vi "Build Instruction List.vi"(6 "Instruction List Starting Offset":u16=2048 format="%04x", 7 "Virtual Memory Unit in":refnum<class "Virtual Memory Unit.lvclass">, 8 "error in (no error)":errorcluster, 11 "Bus Controller in":refnum<class "Bus Controller.lvclass">) -> (0 "error out":errorcluster, 3 "Bus Controller out":refnum<class "Bus Controller.lvclass">, 4 "Instruction List Final Address":u16=2048 format="%04x", 5 "Virtual Memory Unit out":refnum<class "Virtual Memory Unit.lvclass">)   [LabVIEW 2020, in "BCI-1553 API.lvlib" / "Bus Controller.lvclass"]
doc: "Builds the entire instruction list that this Bus Controller will usefor data transactions. The Major Frame must be configured and constructed correctly for this procedure to operate as intended."
uses:
  Bus Controller.lvclass
  Dependencies/Virtual Memory Unit/Virtual Memory Unit.lvclass
  Bus Controller.lvclass/Bus Controller.ctl
  Frames & Messages/Major Frame/Major Frame.lvclass
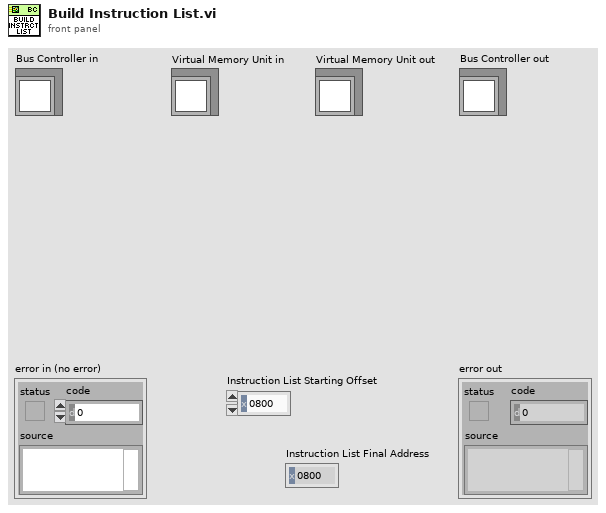
[diagram p1: front panel]
types:
  T1 = cluster{"HP Async Check Addresses":u16[], "HP Async Control Addresses":u16[], "HP Async Data Addresses":u16[], "LP Async Check Addresses":u16[], "LP Async Control Addresses":u16[], "LP Async Data Addresses":u16[]}
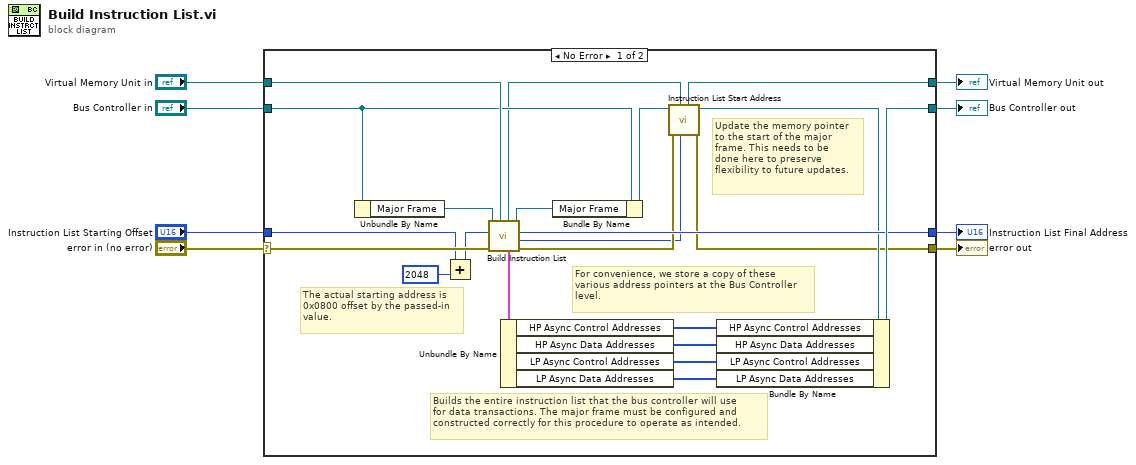
[diagram p0: block diagram]
diagram:
  n1 = case shown="No Error" "error in (no error)" {
    selector: "error in (no error)" -> [w26 w34]
    tunnel: [w15 w34] -> w7
    tunnel: [w20 w33] -> w5
    tunnel: "Bus Controller in" -> [w27 w33]
    tunnel: "Virtual Memory Unit in" -> [w29 w32]
    tunnel: [w12 w32] -> w3
    tunnel: "Instruction List Starting Offset" -> [w10 w31]
    tunnel: [w19 w31] -> w1
    frame No Error {
      # "The actual starting address is\n0x0800 offset by the passed-in\nvalue."
      # "Update the memory pointer\nto the start of the major\nframe. This needs to be\ndone here to preserve\nflexibility to future updates."
      # "For convenience, we store a copy of these\nvarious address pointers at the Bus Controller\nlevel."
      # "Builds the entire instruction list that the bus controller will use\nfor data transactions. The major frame must be configured and\nconstructed correctly for this procedure to operate as intended."
      n2 = Unbundle By Name(w27) -> ("Major Frame"=w30:refnum<class "Major Frame.lvclass">)
      n3 = Add(x=w10, y=u16 2048) -> (x+y=w9:u16)
      n4 = call-dynamic "Build Instruction List.vi"("Virtual Memory Unit in"=w29, "error in (no error)"=w26, "Starting Address"=w9, "Major Frame in"=w30) -> ("error out"=w16:errorcluster, "Instruction List Starting Address"=w14:u16, "Next Available Address"=w19:u16, "Major Frame out"=w28:refnum<class "Major Frame.lvclass">, "Async Pointers"=w25:T1, "Virtual Memory Unit out"=w13:refnum<class "Virtual Memory Unit.lvclass">)  [unwired: 2 in]
      n5 = Unbundle By Name(w25) -> ("HP Async Control Addresses"=w24:u16[], "HP Async Data Addresses"=w23:u16[], "LP Async Control Addresses"=w22:u16[], "LP Async Data Addresses"=w21:u16[])
      n6 = Bundle By Name(cluster=w27, "Major Frame"=w28) -> (w18:refnum<class "Bus Controller.lvclass">)
      n7 = call "Instruction List Start Address.vi"("Starting Address Offset"=w14, "Virtual Memory Unit in"=w13, "error in (no error)"=w16, "Bus Controller in"=w18) -> ("error out"=w15:errorcluster, "Bus Controller out"=w17:refnum<class "Bus Controller.lvclass">, "Virtual Memory Unit out"=w12:refnum<class "Virtual Memory Unit.lvclass">)  [unwired: 5 in]
      n8 = Bundle By Name(cluster=w17, "HP Async Control Addresses"=w24, "HP Async Data Addresses"=w23, "LP Async Control Addresses"=w22, "LP Async Data Addresses"=w21) -> (w20:refnum<class "Bus Controller.lvclass">)
    }
    frame Error {
    }
  }
  "error out" <- w7
  "Bus Controller out" <- w5
  "Virtual Memory Unit out" <- w3
  "Instruction List Final Address" <- w1
